vi "Read iSpkEn.vi"(8 "error in (no error)":errorcluster, 11 "Set iSpkEn MSG in":refnum<class "Set iSpkEn MSG.lvclass">) -> (0 "error out":errorcluster, 2 "iSpkEn":bool[](array[boolean]), 3 "Set iSpkEn MSG out":refnum<class "Set iSpkEn MSG.lvclass">)   [LabVIEW 2014, in "ePAS Library.lvlib" / "Set iSpkEn MSG.lvclass"]
uses:
  Set iSpkEn MSG.lvclass
  Set iSpkEn MSG.lvclass/Set iSpkEn MSG.ctl
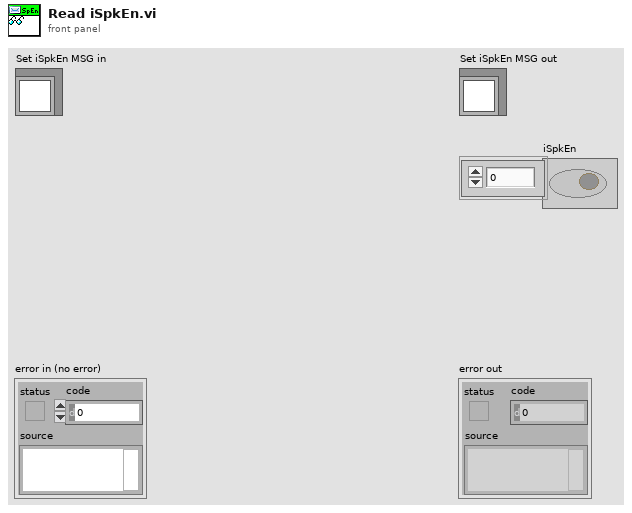
[diagram p1: front panel]
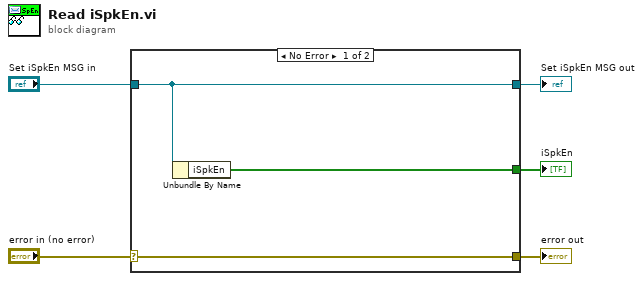
[diagram p0: block diagram]
diagram:
  n1 = case shown="No Error" "error in (no error)" {
    selector: "error in (no error)" -> [w8 w9]
    tunnel: [w8 w9] -> w4
    tunnel: [w7 w10] -> w2
    tunnel: "Set iSpkEn MSG in" -> [w7 w10]
    tunnel: [w6 _] -> w1
    frame No Error {
      n2 = Unbundle By Name(w7) -> ("iSpkEn"=w6:bool[])
    }
    frame Error {
    }
  }
  "error out" <- w4
  "Set iSpkEn MSG out" <- w2
  "iSpkEn" <- w1
